vi "Read Card #.vi"(8 "error in (no error)":errorcluster, 11 "1600 Card Actor in":refnum<class "1600 Card Actor.lvclass">) -> (0 "error out":errorcluster, 2 "Card #":dbl, 3 "1600 Card Actor out":refnum<class "1600 Card Actor.lvclass">)   [LabVIEW 2012, in "Universal Power Meter.lvlib" / "WT1600.lvlib" / "1600Card.lvlib" / "1600 Card Actor.lvclass"]
uses:
  1600 Card Actor.lvclass
  1600 Card Actor.lvclass/1600 Card Actor.ctl
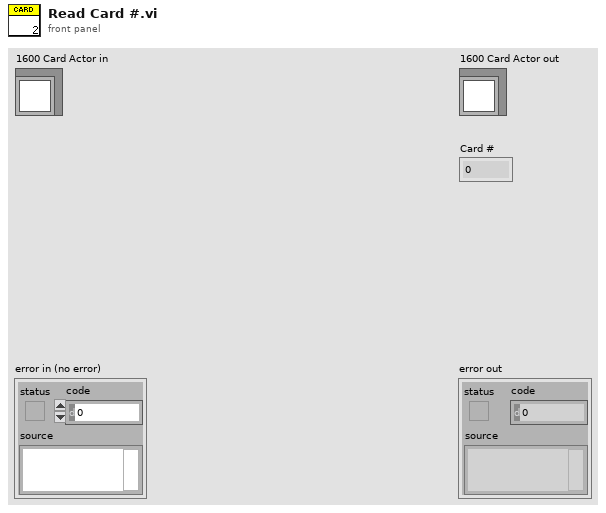
[diagram p1: front panel]
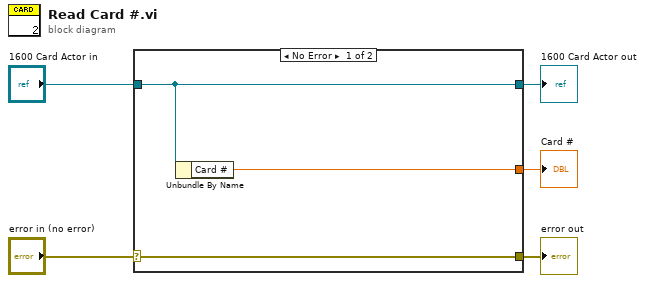
[diagram p0: block diagram]
diagram:
  n1 = case shown="No Error" "error in (no error)" {
    selector: "error in (no error)" -> [w8 w9]
    tunnel: [w8 w9] -> w4
    tunnel: [w7 w10] -> w2
    tunnel: "1600 Card Actor in" -> [w7 w10]
    tunnel: [w6 _] -> w1
    frame No Error {
      n2 = Unbundle By Name(w7) -> ("Card #"=w6:dbl)
    }
    frame Error {
    }
  }
  "error out" <- w4
  "1600 Card Actor out" <- w2
  "Card #" <- w1
